vi "store_user_comments.vi"(8 "error in (no error)":errorcluster, 10 "user comments in":string, 11 "ErrorController in":refnum<class "ErrorController.lvclass">) -> (0 "error out":errorcluster, 3 "ErrorController out":refnum<class "ErrorController.lvclass">)   [LabVIEW 2010, in "ErrorController.lvclass"]
uses:
  ErrorController.lvclass
  ErrorController.lvclass/ErrorController.ctl
  <vilib>/Utility/file.llb/Write To Spreadsheet File (string).vi
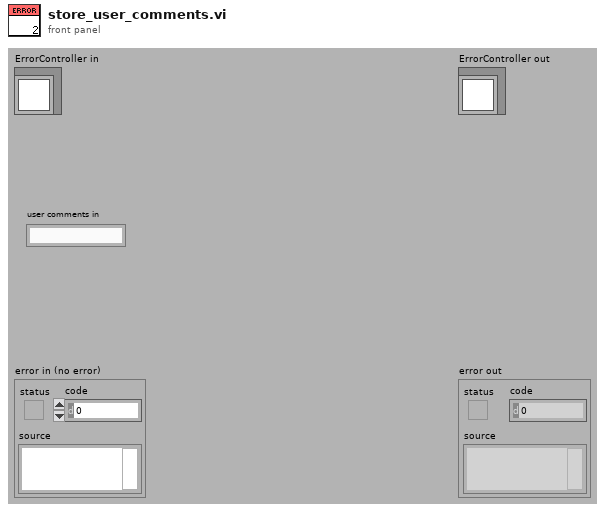
[diagram p1: front panel]
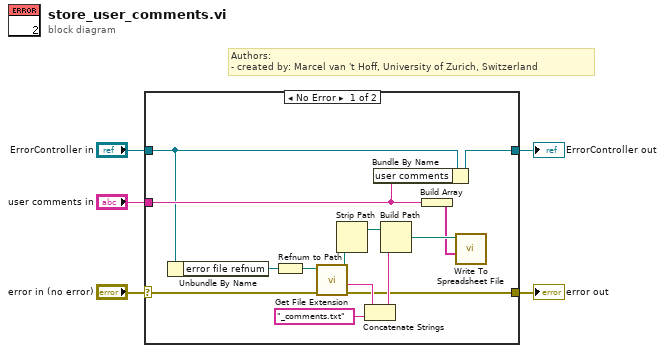
[diagram p0: block diagram]
diagram:
  # "Authors: \n- created by: Marcel van 't Hoff, University of Zurich, Switzerland"
  n1 = case shown="No Error" "error in (no error)" {
    selector: "error in (no error)" -> [w11 w21]
    tunnel: [w10 w21] -> w4
    tunnel: [w19 w20] -> w2
    tunnel: "ErrorController in" -> [w6 w20]
    tunnel: "user comments in" -> [w8 _]
    frame No Error {
      n2 = Unbundle By Name(w6) -> ("error file refnum"=w18:refnum<file>)
      n3 = Refnum to Path(1:w18) -> (0:w17:path)
      n4 = call <vilib>:"Get File Extension.vi"("error in (no error)"=w11, "file"=w17) -> ("error out"=w10:errorcluster, "filename without extension"=w15:string, "dup file"=w16:path)  [unwired: 6 in, 1 out]
      n5 = Strip Path(path=w16) -> (stripped path=w13:path)  [unwired: 1 out]
      n6 = Concatenate Strings(w15, "_comments.txt" ("string")) -> (w12:string)
      n7 = Bundle By Name(cluster=w6, "user comments"=w8) -> (w19:refnum<class "ErrorController.lvclass">)
      n8 = Build Path(base path=w13, name or relative path=w12) -> (appended path=w9:path)
      n9 = Build Array(w8) -> (w7:string[])
      n10 = call-poly <vilib>:"Write To Spreadsheet File.vi"("1D data"=w7, "file path (dialog if empty)"=w9) -> ()  [unwired: 6 in, 1 out]
    }
    frame Error {
    }
  }
  "error out" <- w4
  "ErrorController out" <- w2
